vi "DAQmx_Pulse_TrainSlow.vi"(0 "Counter(s)":tag="PXI1Slot2/ctr0", 1 "Start?":bool=TRUE, 3 "HighTime":dbl=20.0 caption="Frequency (Hz)" format="%0.2f", 5 "LowTime":dbl=1.0 caption="Duty Cycle" min=0.0 format="%0.2f") -> ()   [LabVIEW 2009]
doc: "I. Description:\nThis example demonstrates how to generate a continuous digital pulse train from a Counter Output Channel. The Frequency, Duty Cycle, and Idle State are all configurable. \n\nThis example shows how to configure the pulse in terms of Frequency/Duty Cycle, but can easily be modified to generate a pulse in terms of Time or Ticks.\n\nII. Instructions for Running:\n1. Select the Physical Channel which corresponds to the counter you want to output your signal to on the DAQ device.\n2. Enter the Frequency and Duty Cycle to define the pulse parameters. You can also change the Idle State to determine the beginning and end states of the output. If the Idle State is High, the generation will use inverted logic. Additionally, you can set the Initial Delay (in seconds) which will delay the beginning of the pulse train from the start call; this is currently wired to 0.0 on the diagram. \nNote: Use the Measure Period example to verify you are outputting the pulse train on the DAQ device.\n\nIII. Block Diagram Steps:\n1. Create an empty task\n2. Create a Counter Output channel to produce a Pulse in terms of Frequency. If the Idle State of the pulse is set to low, the state of the line will begin low and remain low after the generation is stopped.\n3. Use the DAQmx Base Timing VI (Implicit) to configure the duration of the pulse generation.\n4. Call the Start VI to arm the counter and begin the pulse train generation.\n5. Loop continuously until the user presses the Stop button. Check for errors every 100 ms using the Is Task Done? VI\n6. Stop the task\n7. Clear the Task.\n\nIV. I/O Connections Overview:\nThe counter will output the pulse train on the output terminal of the counter specified in the Physical Channel I/O control. \n\nIn this example the output will be sent to the default output terminal on ctr0.\n\nFor more information on the default counter input and output terminals for your device, open the NI-DAQmx Help, and refer to Counter Signal Connections found under the Device Considerations book in the table of contents."
uses:
  <vilib>/DAQmx/configure/timing.llb/DAQmx Timing (Implicit).vi
  <vilib>/DAQmx/create/channels.llb/DAQmx Create Channel (CO-Pulse Generation-Time).vi
panel:
  out "error out":errorcluster
  # "For instructions, select Help>>Show Context Help"
  # "Channel Parameters"
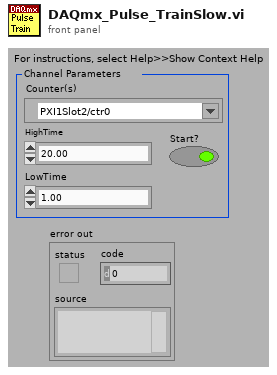
[diagram p1: front panel]
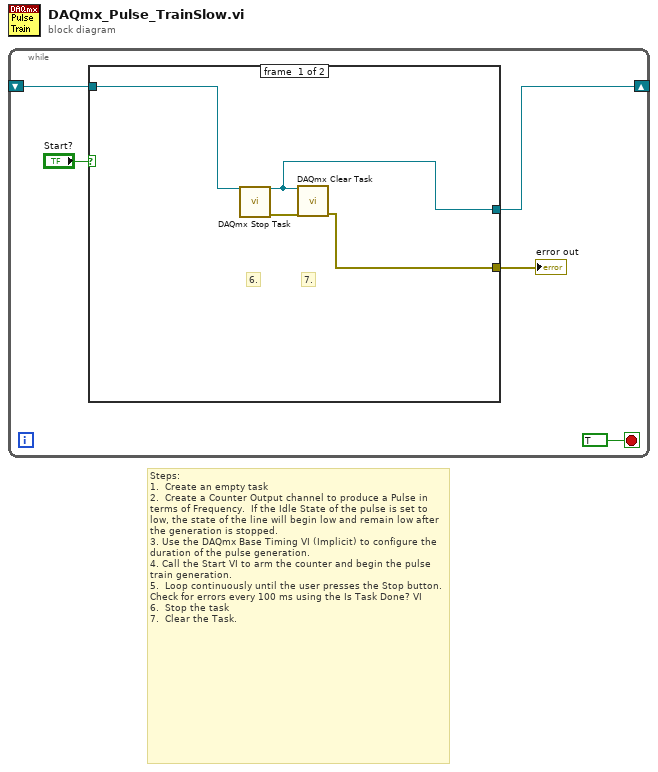
[diagram p0: block diagram]
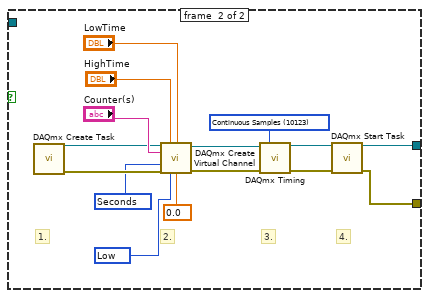
[diagram p2: hidden frame]
diagram:
  # "Steps: \n1.  Create an empty task\n2.  Create a Counter Output channel to produce a Pulse in terms of Frequency.  If the Idle State of the pulse is set to low, the state of the line will begin low and remain low after the generation is stopped.\n3. Use the DAQmx Base Timing VI (Implicit) to configure the duration of the pulse generation.\n4. Call the Start VI to arm the counter and begin the pulse train generation.\n5.  Loop continuously until the user presses the Stop button. Check for errors every 100 ms using the Is Task Done? VI\n6.  Stop the task\n7.  Clear the Task."
  n1 = while {
    shift-right: [w5] -> _
    shift-left: _ -> [w3]
    stop <- TRUE stop-if-true
    n2 = case shown="True" "Start?" {
      tunnel: [w7 w13] -> w5
      tunnel: w3 -> [w8 _]
      tunnel: [w6 w10] -> w1
      frame #0 {
        # "7."
        # "6."
        n3 = call <vilib>:"DAQmx Stop Task.vi"("task/channels in"=w8) -> ("task out"=w7:refnum<k21>, "error out"=w9:errorcluster)  [unwired: 1 in, 12 out]
        n4 = call <vilib>:"DAQmx Clear Task.vi"("task in"=w7, "error in"=w9) -> ("error out"=w6:errorcluster)  [unwired: 13 out]
      }
      frame #1 {
        w11 = 10214 items=["High"=10192, "Low"=10214] ("idle state")
        w12 = 10364 items=["Seconds"=10364] ("units")
        w20 = 10123 items=["Finite Samples"=10178, "Continuous Samples"=10123] ("sample mode")
        # "4."
        # "3."
        # "2."
        # "1."
        n5 = call <vilib>:"DAQmx Create Task.vi"() -> ("task out"=w14:refnum<k21>, "error out"=w15:errorcluster)  [unwired: 5 in, 9 out]
        n6 = call-poly <vilib>:"DAQmx Create Virtual Channel.vi"("task in"=w14, "high time"="HighTime", "low time"="LowTime", "counter"="Counter(s)", "units"=w12, "error in"=w15, "idle state"=w11, "initial delay"=0.0) -> ("task out"=w23:refnum<k21>, "error out"=w24:errorcluster)  [unwired: 1 in, 5 out]
        n7 = call-poly <vilib>:"DAQmx Timing.vi"("task/channels in"=w23, "sample mode"=w20, "error in"=w24) -> ("task out"=w21:refnum<k21>, "error out"=w22:errorcluster)  [unwired: 1 in, 10 out]
        n8 = call <vilib>:"DAQmx Start Task.vi"("task/channels in"=w21, "error in"=w22) -> ("task out"=w13:refnum<k21>, "error out"=w10:errorcluster)  [unwired: 12 out]
      }
    }
    "error out" <- w1
  }
